vi "Get snmp Item(s).vi"(5 "UDP Port":u16=161, 6 "timeout ms (25000)":i32=25000, 7 "IP Address of SNMP Device":string="10.211.1.231", 8 "error in (no error)":errorcluster, 9 "OID ARRAY":string[](array[string]), 10 "Community Name":string="public", 11 "connection ID in":refnum<k16>) -> (0 "error out":errorcluster, 1 "error-string":string, 2 "SnmpDataAsStrings":string[][](array[string]), 3 "connection ID out":refnum<k16>, 4 "error-status":u8)   [LabVIEW 2017]
doc: "This VI is used to perform a basic GET request from a specified agent. The VI requires an array of OID values to be retrieved from the agent. It will return a 2D array of strings containing containing an ASCII representation of an OID/TYPE/VALUE which was returned from the agent."
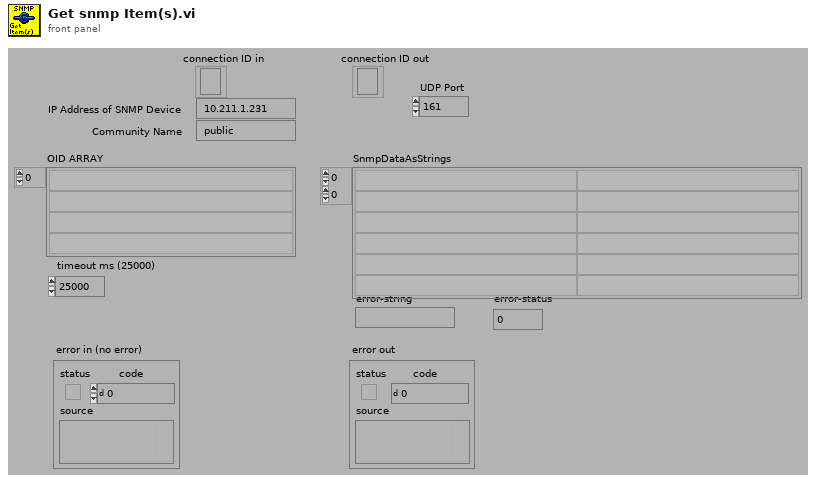
[diagram p1: front panel]
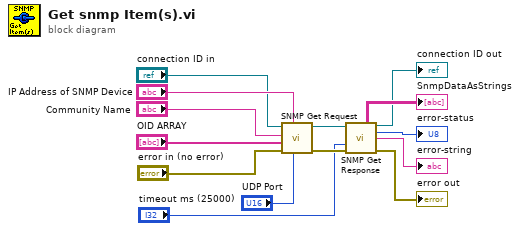
[diagram p0: block diagram]
diagram:
  n1 = call "SNMP Get Request.vi"("UDP Port"="UDP Port", "IP Address"="IP Address of SNMP Device", "error in (no error)"="error in (no error)", "OID ARRAY"="OID ARRAY", "Community Name"="Community Name", "connection ID"="connection ID in") -> ("error out"=w6:errorcluster, "connection ID"=w7:refnum<k16>)  [unwired: 4 out]
  n2 = call "SNMP Get Response.vi"("connection ID"=w7, "timeout ms (25000)"="timeout ms (25000)", "error in (no error)"=w6) -> ("SnmpDataAsStrings"=→"SnmpDataAsStrings":string[][], "connection ID out"=→"connection ID out":refnum<k16>, "error-status"=→"error-status":i32, "error-string"=→"error-string":string, "error out"=→"error out":errorcluster)  [unwired: 8 out]
